vi "pannel-to-devicelist.vi"(11 "pannel-list":T4(array[cluster])=[{"node"=[{"ID"="1", "Attribute"="dev", "Action"="", "name"="台灯"}, {"ID"="2", "Attribute"="dev", "Action"="bright-gear", "name"="阅读灯"}], "ID"="0"}, {"node"=[{"ID"="1", "Attribute"="dev", "Action"="", "name"="顶灯"}, {"ID"="2", "Attribute"="dev", "Action"="", "name"="台灯"}], "ID"="1"}, {"node"=[{"ID"="1", "Attribute"="dev", "Action"="open", "name"="窗帘"}, {"ID"="2", "Attribute"="dev", "Action"="close", "name"="窗帘"}], "ID"="2"}]) -> (3 "device-list out":T1(array[cluster]))   [LabVIEW 2019]
panel:
  in  "device-list":T1(array[cluster])
  in  "device":T2
  in  "info":T3
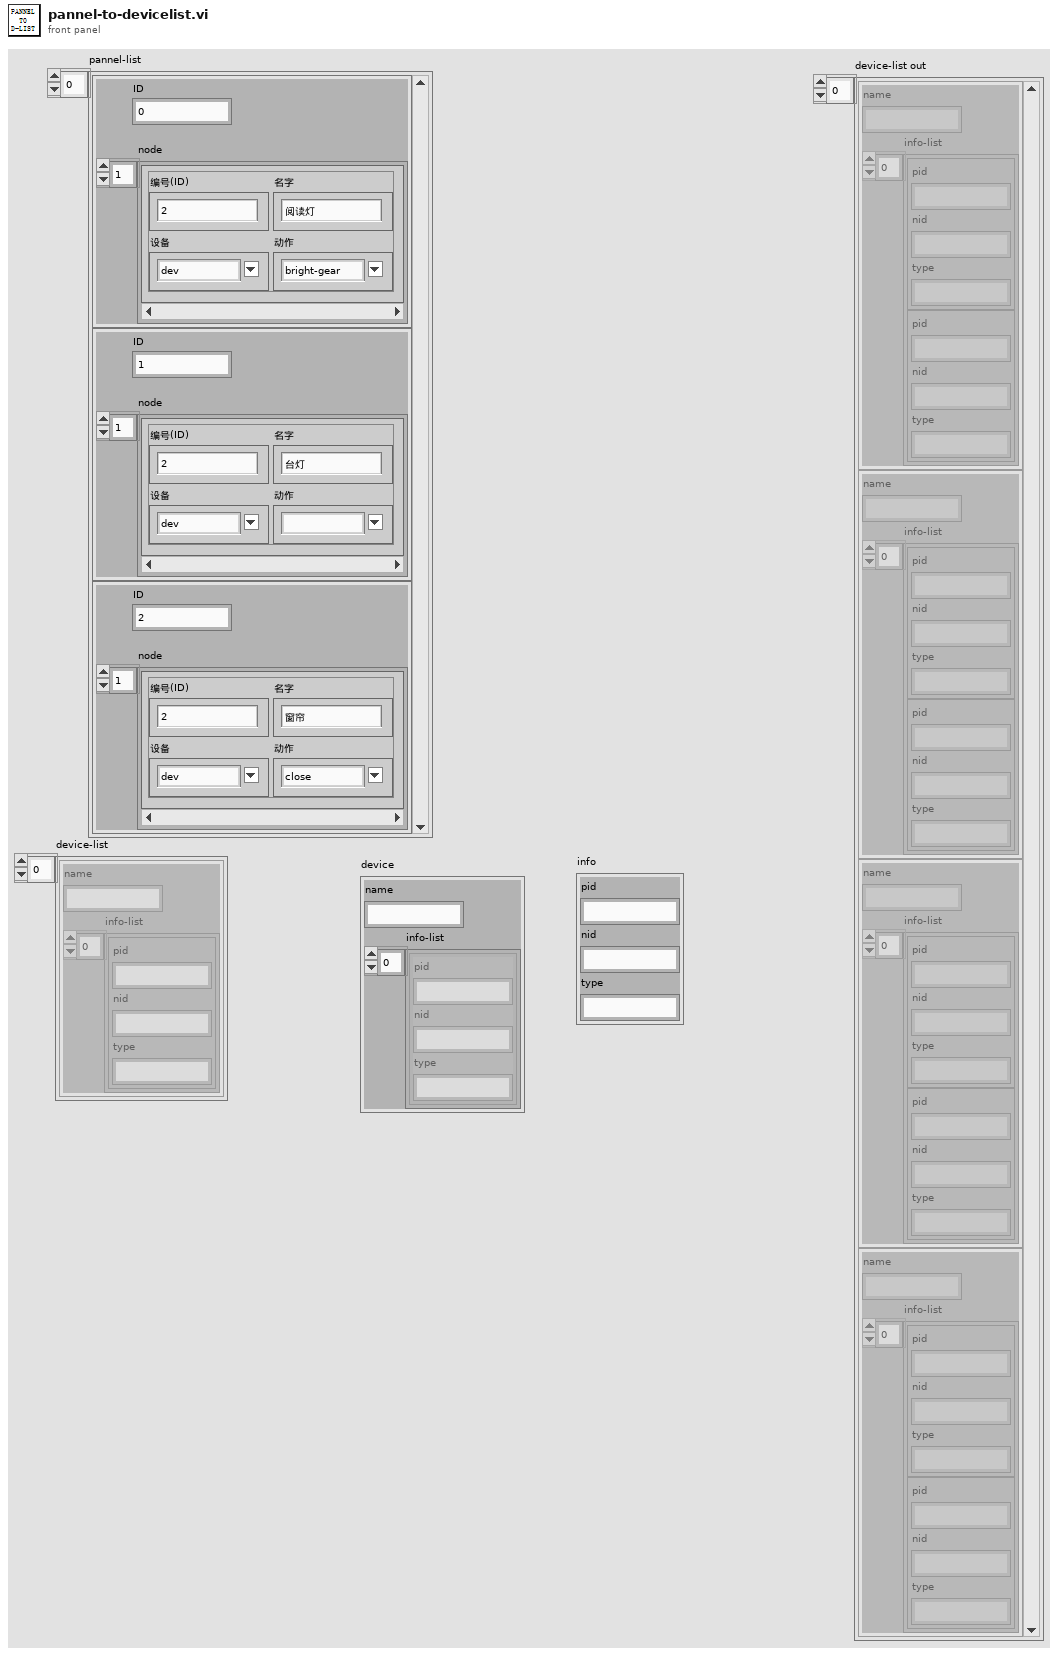
[diagram p1: front panel]
types:
  T1 = cluster{"name":string, "info-list":cluster{"pid":string, "nid":string, "type":string}[]}[]
  T2 = cluster{"name":string, "info-list":cluster{"pid":string, "nid":string, "type":string}[]}
  T3 = cluster{"pid":string, "nid":string, "type":string}
  T4 = cluster{"node":cluster{"ID":string, "Attribute":string, "Action":string, "name":string}[], "ID":string}[]
  T5 = cluster{"ID":string, "Attribute":string, "Action":string, "name":string}[]
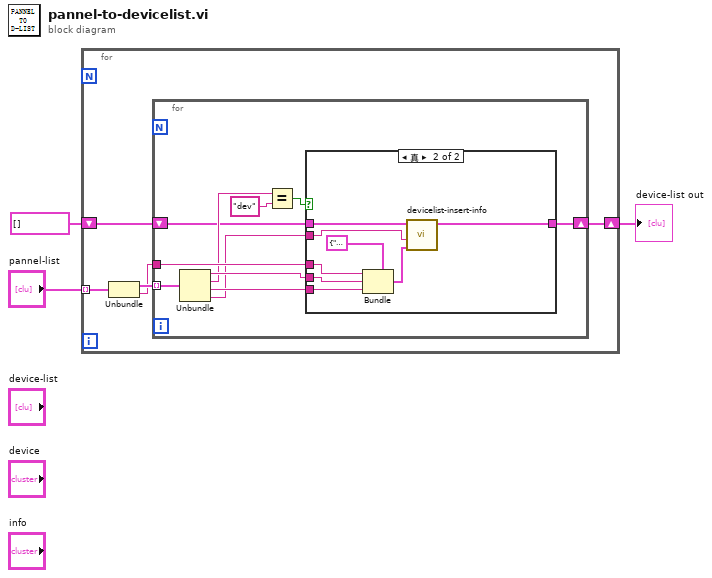
[diagram p0: block diagram]
diagram:
  n1 = for {
    tunnel: "pannel-list" -> [w8] mode=indexing
    shift-right: [w4] -> w2
    shift-left: T1 [] ("device-list output") -> [w5]
    n2 = Unbundle(w8) -> ("node"=w7:T5, "ID"=w6:string)
    n3 = for {
      tunnel: w7 -> [w18] mode=indexing
      tunnel: w6 -> [w17]
      shift-right: [w9] -> w4
      shift-left: w5 -> [w10]
      n4 = Unbundle(w18) -> ("ID"=w16:string, "Attribute"=w13:string, "Action"=w15:string, "name"=w14:string)
      n5 = Equal?(x=w13, y="dev") -> (x = y?=w11:bool)
      n6 = case shown="真" w11 {
        tunnel: w17 -> [_ w25]
        tunnel: w16 -> [_ w24]
        tunnel: w15 -> [_ w23]
        tunnel: w14 -> [_ w22]
        tunnel: w10 -> [w19 w21]
        tunnel: [w19 w20] -> w9
        frame False {
        }
        frame True {
          n7 = Bundle(cluster=T3 {"pid"="", "nid"="", "type"=""} ("info"), "pid"=w25, "nid"=w24, "type"=w23) -> (w26:T3)
          n8 = call "devicelist-insert-info.vi"("info"=w26, "name"=w22, "device-list"=w21) -> ("device-list output"=w20:T1)  [unwired: 8 in]
        }
      }
    }
  }
  "device-list out" <- w2
